vi "Write.vi"(8 "error in (no error)":errorcluster, 10 "Data":string, 11 "Instrument Interface in":refnum<class "Instrument.lvclass">) -> (0 "error out":errorcluster, 3 "Instrument Interface out":refnum<class "Instrument.lvclass">)   [LabVIEW 2020, in "Low Level PSU With Tests.lvlib" / "Instrument.lvclass"]
uses:
  Instrument.lvclass
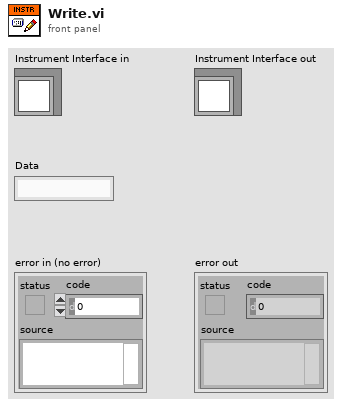
[diagram p1: front panel]
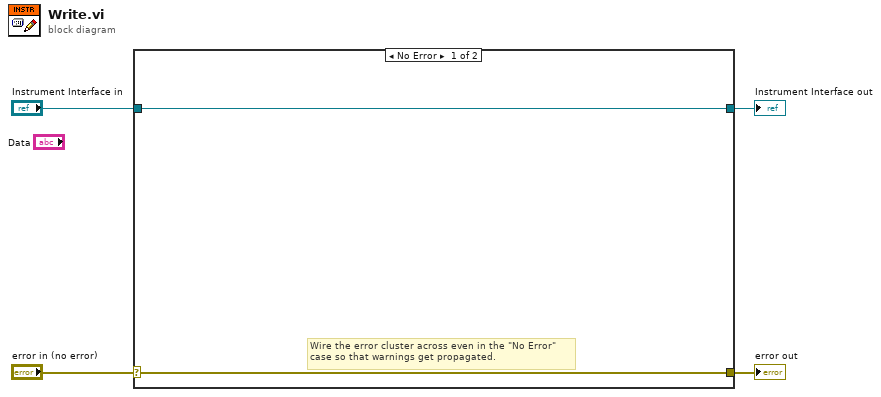
[diagram p0: block diagram]
diagram:
  n1 = case shown="No Error" "error in (no error)" {
    selector: "error in (no error)" -> [w5 w8]
    tunnel: [w5 w8] -> w3
    tunnel: [w6 w7] -> w1
    tunnel: "Instrument Interface in" -> [w6 w7]
    frame No Error {
      # "Wire the error cluster across even in the \"No Error\"\ncase so that warnings get propagated."
    }
    frame Error {
    }
  }
  "error out" <- w3
  "Instrument Interface out" <- w1
